vi "DIAdem Process Stop Request.vi"(5 "error in (no error)":errorcluster, 7 "DIAdem Queue":T1, 8 "DIAdem Reference":T3) -> (0 "error out":errorcluster, 2 "Script Result":string, 3 "DIAdem Reference":T3)   [LabVIEW 2011]
uses:
  <vilib>/ExportToExcel/DIAdem Reference.ctl
  DIAdem Daemon Queue.ctl
  DIAdem Daemon Script Type.ctl
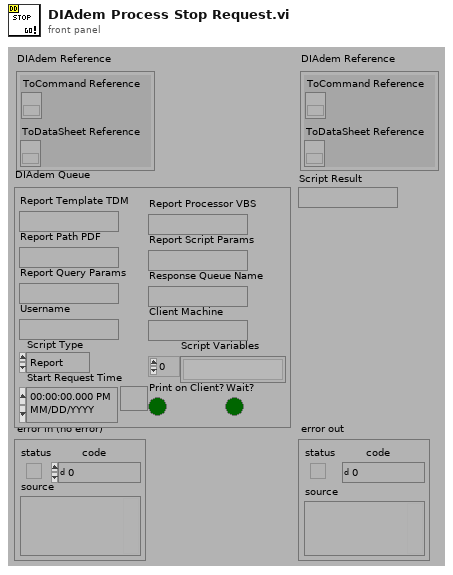
[diagram p1: front panel]
types:
  T1 = typedef "DIAdem Daemon Queue.ctl" = cluster{"Report Template TDM":path, "Report Processor VBS":path, "Report Path PDF":path, "Report Script Params":string, "Username":string, "Script Type":T2, "Report Query Params":string, "Client Machine":string, "Print on Client?":bool, "Response Queue Name":string, "Script Variables":string[], "Start Request Time":timestamp, "Wait?":bool}
  T2 = typedef "DIAdem Daemon Script Type.ctl" = enum16{"Report", "Query", "Script", "Datasheet", "Append", "Restart", "Stop"}
  T3 = typedef "DIAdem Reference.ctl" = cluster{"ToCommand Reference":refnum<k7>, "ToDataSheet Reference":refnum<k7>}
  T4 = cluster{"ToCommand Reference":bool, "ToDataSheet Reference":bool}
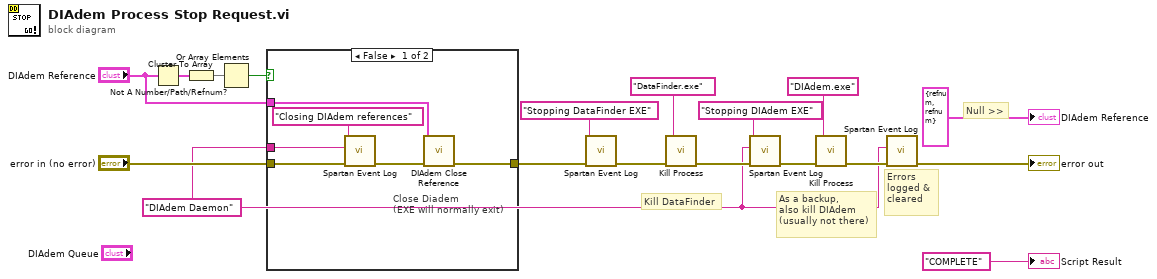
[diagram p0: block diagram]
diagram:
  w1 = "DIAdem Daemon"
  # "As a backup,\nalso kill DIAdem\n(usually not there)"
  # "Kill DataFinder"
  # "Errors\nlogged &\ncleared"
  # "Null >>"
  n1 = Not A Number/Path/Refnum?(number/path/refnum="DIAdem Reference") -> (NaN/Path/Refnum?=w16:T4)
  n2 = Cluster To Array(cluster=w16) -> (array=w17:bool[])
  n3 = Or Array Elements(Boolean array=w17) -> (logical OR=w18:bool)
  n4 = case shown="False" w18 {
    tunnel: "error in (no error)" -> [w23 w25]
    tunnel: [w20 w25] -> w3
    tunnel: "DIAdem Reference" -> [w24 _]
    tunnel: w1 -> [w19 _]
    frame False {
      # "Close Diadem\n(EXE will normally exit)"
      n5 = call "Spartan Event Log.vi"("error in (no error)"=w23, "module (\"\")"=w19, "message (\"\")"="Closing DIAdem references") -> ("error out"=w22:errorcluster)  [unwired: 2 in, 3 out]
      n6 = call <vilib>:"DIAdem Close Reference.vi"("error in (no error)"=w22, "DIAdem Reference"=w24) -> ("error out"=w20:errorcluster)  [unwired: 9 out]
    }
    frame True {
      # "<< Null incoming ref?  nothing to stop"
    }
  }
  n7 = call "Spartan Event Log.vi"("error in (no error)"=w3, "message (\"\")"="Stopping DataFinder EXE") -> ("error out"=w9:errorcluster)  [unwired: 3 in, 3 out]
  n8 = call "Kill Process.vi"("error in (no error)"=w9, "Name of Process to kill (\"\")"="DataFinder.exe" ("Name of Process to kill (\"\")")) -> ("error out"=w10:errorcluster)  [unwired: 5 out]
  n9 = call "Spartan Event Log.vi"("error in (no error)"=w10, "module (\"\")"=w1, "message (\"\")"="Stopping DIAdem EXE") -> ("error out"=w7:errorcluster)  [unwired: 2 in, 3 out]
  n10 = call "Kill Process.vi"("error in (no error)"=w7, "Name of Process to kill (\"\")"="DIAdem.exe" ("Name of Process to kill (\"\")")) -> ("error out"=w11:errorcluster)  [unwired: 5 out]
  n11 = call "Spartan Event Log.vi"("error in (no error)"=w11, "module (\"\")"=w1) -> ("error out"=→"error out":errorcluster)  [unwired: 3 in, 3 out]
  "DIAdem Reference" <- T3 {"ToCommand Reference"=refnum, "ToDataSheet Reference"=refnum} ("DIAdem Reference")
  "Script Result" <- "COMPLETE" ("Script Result")
